vi "Fetch Waveform.vi"(1 "Custom Source ID":string, 4 "Sparsing (0: Every point)":i32, 5 "Number of points (0: All points)":i32, 6 "Segment number (0: All segment)":i16, 7 "First point (0: First point)":i32, 8 "error in (no error)":errorcluster, 9 "Timeout (10000 ms)":u32=10000, 10 "Source (0: Channel 1)":u16(ring) items=["Channel 1", "Channel 2", "Channel 3", "Channel 4", "Memory 1", "Memory 2", "Memory 3", "Memory 4", "Function 1", "Function 2", "Function 3", "Function 4", "Function 5", "Function 6", "Function 7", "Function 8", "Other"], 11 "VISA resource name":refnum<visa-resource-name>) -> (0 "error out":errorcluster, 2 "Waveform Graph":waveform(dbl)(graph), 3 "VISA resource name out":refnum<visa-resource-name>)   [LabVIEW 2013, in "LeCroy Wave Series.lvlib"]
doc: "Returns the waveform the oscilloscope acquired for the specified channel. The waveform is from an acquisition that you initiate prior to calling this VI.\n\nYou use the Initiate VI to start an acquisition on the channels that you enable with the <B>Configure Channel</B> VI. The oscilloscope acquires waveforms for the enabled channels concurrently. You must call this VI separately for each enabled channel to obtain the waveforms.\n\nYou can call the <B>lcwave Read Single Waveform</B> VI or <B>lcwave Read Multiple Waveforms</B> VI instead of using low level VIs.\n\n<B>Note</B> This VI does not check the instrument status. Typically, you call this VI only in a sequence of calls to other low-level instrument driver VIs. The sequence performs one operation. You use the low-level VIs to optimize one or more aspects of interaction with the instrument."
uses:
  LeCroy Wave Series.lvlib
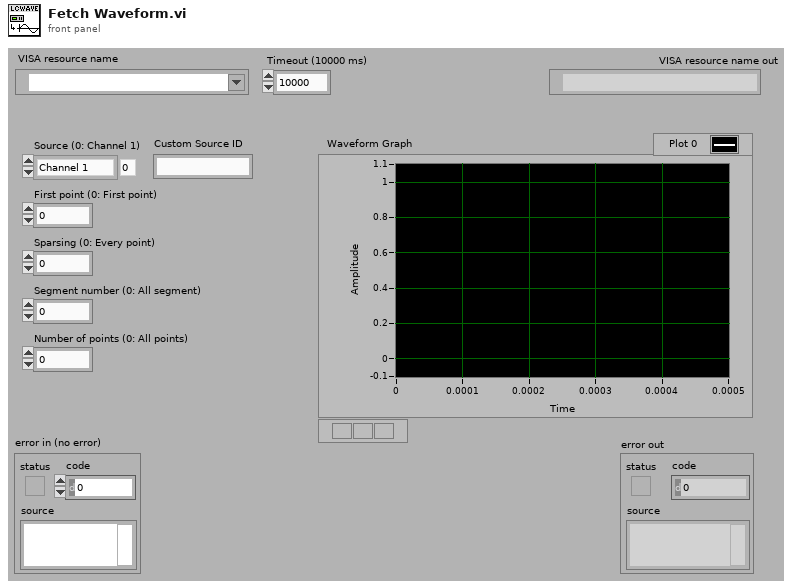
[diagram p1: front panel]
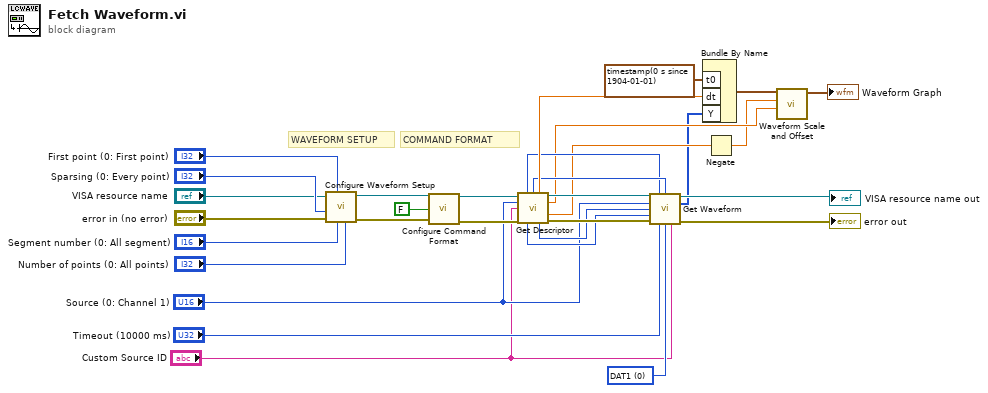
[diagram p0: block diagram]
diagram:
  w20 = u16 0 items=["DAT1", "DAT2"] ("Array (1: DAT1)")
  # "WAVEFORM SETUP"
  # "COMMAND FORMAT"
  n1 = call "Configure Waveform Setup.vi"("Number of points (0: All points)"="Number of points (0: All points)", "Segment number (0: All segment)"="Segment number (0: All segment)", "First point (0: First point)"="First point (0: First point)", "error in (no error)"="error in (no error)", "Sparsing (0: Every point)"="Sparsing (0: Every point)", "VISA resource name"="VISA resource name") -> ("error out"=w25:errorcluster, "VISA resource name out"=w26:refnum<visa-resource-name>)  [unwired: 4 in]
  n2 = call "Configure Command Format.vi"("VISA resource name"=w26, "Command format (T: Byte)"=FALSE, "error in (no error)"=w25) -> ("VISA resource name out"=w18:refnum<visa-resource-name>, "error out"=w17:errorcluster)  [unwired: 11 in]
  n3 = call "Get Descriptor.vi"("VISA resource name"=w18, "Source (0: Channel 1)"="Source (0: Channel 1)", "Custom Source ID"="Custom Source ID", "error in (no error)"=w17) -> ("First Valid Point"=w14:i32, "Last Valid Point"=w15:i32, "Horizontal interval"=w21:sgl, "VISA resource name out"=w31:refnum<visa-resource-name>, "Vertical gain"=w11:sgl, "Vertical offset"=w10:sgl, "Number Of Data Points"=w19:i32, "Command type"=w27:i16, "error out"=w30:errorcluster)  [unwired: 1 in, 2 out]
  n4 = call "Get Waveform.vi"("VISA resource name"=w31, "First Valid Point"=w14, "Last Valid Point"=w15, "Source (0: Channel 1)"="Source (0: Channel 1)", "Command type (0: byte)"=w27, "Number Of Data Points (10000)"=w19, "error in (no error)"=w30, "Timeout (10000 ms)"="Timeout (10000 ms)", "Array (0: DAT1)"=w20, "Custom Source ID"="Custom Source ID") -> ("VISA resource name out"=→"VISA resource name out":refnum<visa-resource-name>, "Waveform Graph"=w4:i16[], "error out"=→"error out":errorcluster)  [unwired: 3 in]
  n5 = Bundle By Name ("Build Waveform")("t0"=timestamp(0 s since 1904-01-01), "dt"=w21, "Y"=w4) -> (w13:waveform(i16))  [unwired: 1 in]
  n6 = Negate(x=w10) -> (-x=w9:sgl)
  n7 = call <vilib>:"Waveform Scale and Offset.vi"("scale"=w11, "offset"=w9, "waveform in"=w13) -> ("waveform out"=→"Waveform Graph":waveform(dbl))  [unwired: 7 in, 1 out]
